vi "Execute.vi"(8 "error in":errorcluster, 11 "Switch Step in":refnum<class "Switch Step.lvclass">) -> (0 "error out":errorcluster, 1 "Next Step?":bool, 2 "MSG":string, 3 "Switch Step out":refnum<class "Switch Step.lvclass">)   [LabVIEW 2018, in "Sequence Composition.lvlib" / "Switch Step.lvclass"]
uses:
  Switch Step.lvclass
  Switch Step.lvclass/Switch Step.ctl
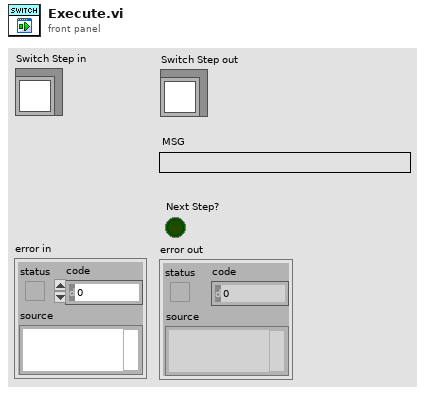
[diagram p1: front panel]
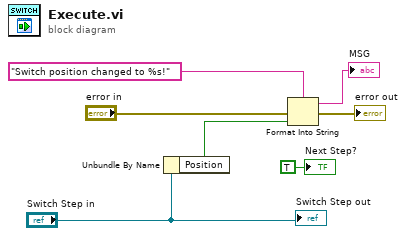
[diagram p0: block diagram]
diagram:
  n1 = Unbundle By Name("Switch Step in") -> ("Position"=w5:bool)
  n2 = Format Into String(format string="Switch position changed to %s!" ("MSG 2"), error in="error in", w5) -> (resulting string=→"MSG":string, error out=→"error out":errorcluster)  [unwired: 1 in]
  "Switch Step out" <- "Switch Step in"
  "Next Step?" <- TRUE ("Next Step?")
